vi "Set heating mode.vi"(8 "error in (no error)":errorcluster, 10 "MODE":enum16{"Precise-Mode", "Fast-Mode"}(ring), 11 "VISA resource name":refnum<visa-resource-name>) -> (0 "error out":errorcluster, 3 "VISA resource name out":refnum<visa-resource-name>)   [LabVIEW 2018]
panel:
  out "resulting string":string
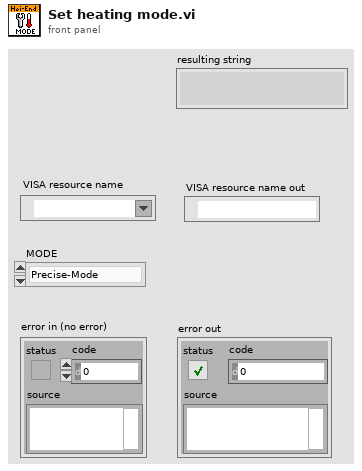
[diagram p1: front panel]
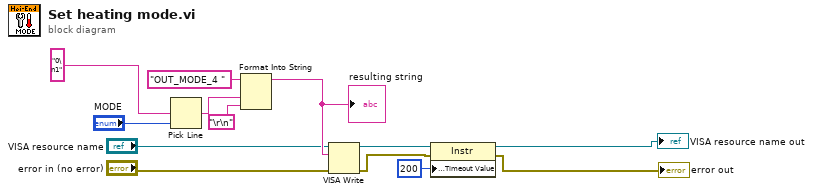
[diagram p0: block diagram]
diagram:
  n1 = Pick Line(multi-line string="0\n1" ("string (\"\")"), line index="MODE") -> (output string=w2:string)  [unwired: 1 in]
  n2 = Format Into String(initial string="OUT_MODE_4 ", w2, "\r\n") -> (resulting string=w12:string)  [unwired: 2 in, 1 out]
  "resulting string" <- w12
  n3 = VISA Write(VISA resource name="VISA resource name", write buffer=w12, error in (no error)="error in (no error)") -> (VISA resource name out=w8:refnum<visa-resource-name>, error out=w7:errorcluster)  [unwired: 1 out]
  n4 = property class="Instr"(reference=w8, error in=w7, "General Settings:Timeout Value"=u32 200) -> (reference out=→"VISA resource name out":refnum<visa-resource-name>, error out=→"error out":errorcluster)
